vi "Pack Step Value.vi"(8 "error in":errorcluster, 10 "Value":string, 11 "Switch Step in":refnum<class "Switch Step.lvclass">) -> (0 "error out":errorcluster, 3 "Switch Step out":refnum<class "Switch Step.lvclass">)   [LabVIEW 2016, in "Sequence Composition.lvlib" / "Switch Step.lvclass"]
uses:
  Switch Step.lvclass
  Switch Step.lvclass/Switch Step.ctl
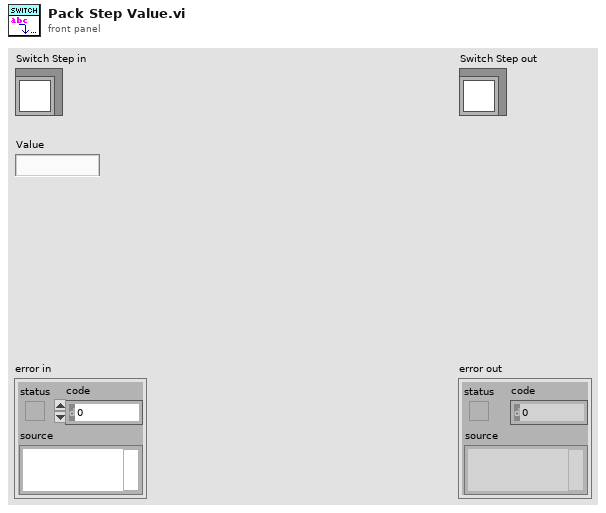
[diagram p1: front panel]
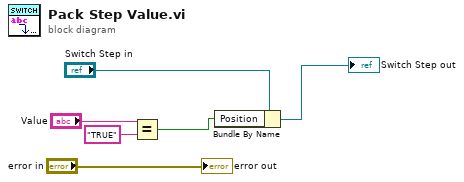
[diagram p0: block diagram]
diagram:
  n1 = Equal?(x="Value", y="TRUE") -> (x = y?=w2:bool)
  n2 = Bundle By Name(cluster="Switch Step in", "Position"=w2) -> (→"Switch Step out":refnum<class "Switch Step.lvclass">)
  "error out" <- "error in"
